vi "Read Configuration Data.vi"(8 "error in":errorcluster) -> (0 "error out":errorcluster, 3 "MHL Configuration":T1)   [LabVIEW 2015]
uses:
  controls/MHL Configuration.ctl
  Boiler System Globals.vi
  <vilib>/Utility/config.llb/NI_LVConfig.lvlib
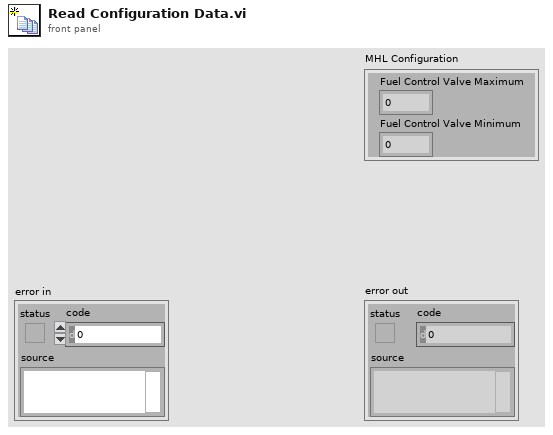
[diagram p1: front panel]
types:
  T1 = typedef "MHL Configuration.ctl" = cluster{"Fuel Control Valve Maximum":dbl, "Fuel Control Valve Minimum":dbl}
  T2 = typedef "NI_LVConfig.lvlib/Config Data RefNum.ctl" = refnum<k1>
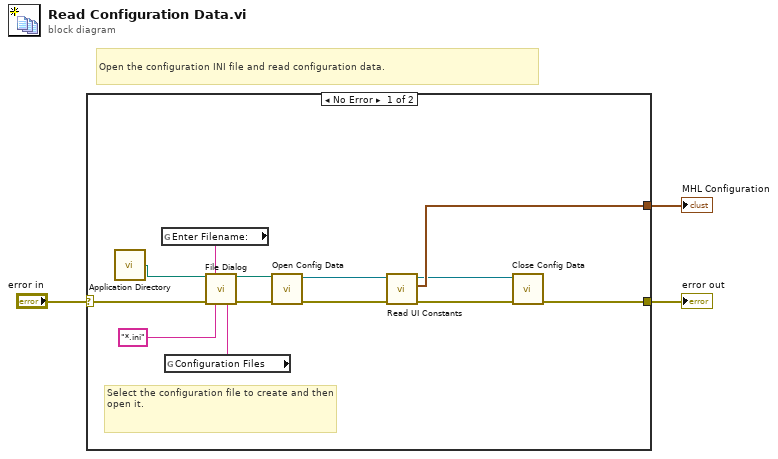
[diagram p0: block diagram]
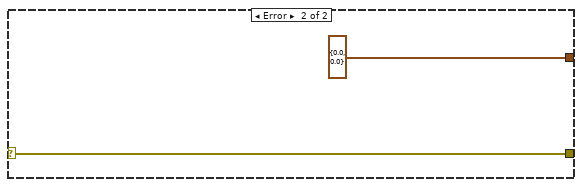
[diagram p2: hidden frame]
diagram:
  # "Open the configuration INI file and read configuration data."
  n1 = case shown="No Error" "error in" {
    selector: "error in" -> [w10 w18]
    tunnel: [w7 w18] -> w3
    tunnel: [w5 T1 {"Fuel Control Valve Maximum"=0.0, "Fuel Control Valve Minimum"=0.0} ("MHL Configuration")] -> w2
    frame No Error {
      # "Select the configuration file to create and then open it."
      n2 = call <vilib>:"Application Directory.vi"() -> ("Application Directory"=w13:path)
      n3 = global read "Boiler System Globals.vi" "Enter Filename:"() -> (w16:string)
      n4 = global read "Boiler System Globals.vi" "Configuration Files"() -> (w14:string)
      n5 = call "File Dialog"("start path"=w13, "prompt"=w16, "error in"=w10, "pattern (all files)"="*.ini", "pattern label"=w14) -> ("selected path"=w11:path, "error out"=w12:errorcluster)  [unwired: 7 in, 2 out]
      n6 = call <vilib>:"Open Config Data.vi"("error in (no error)"=w12, "configuration file path"=w11) -> ("error out"=w8:errorcluster, "refnum"=w9:T2)  [unwired: 1 in, 7 out]
      n7 = call "Read UI Constants.vi"("error in"=w8, "CFG File Refnum in"=w9) -> ("error out"=w6:errorcluster, "MHL Configuration"=w5:T1, "CFG File Refnum out"=w4:T2)  [unwired: 7 in]
      n8 = call <vilib>:"Close Config Data.vi"("error in (no error)"=w6, "refnum"=w4) -> ("error out"=w7:errorcluster)  [unwired: 1 in, 8 out]
    }
    frame Error {
    }
  }
  "error out" <- w3
  "MHL Configuration" <- w2
